vi "Time Shift.vi"(9 "Numeric":i32, 11 "Graph in":cluster{dbl[], dbl[]}) -> (3 "Graph out":cluster{dbl[], dbl[]})   [LabVIEW 2015]
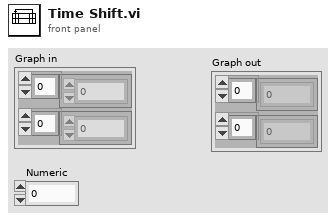
[diagram p1: front panel]
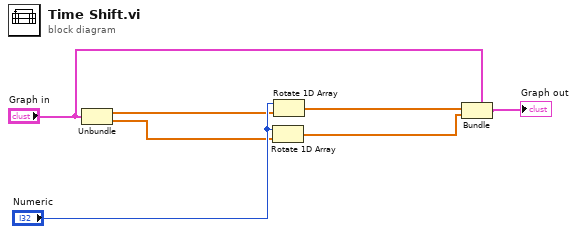
[diagram p0: block diagram]
diagram:
  n1 = Unbundle("Graph in") -> (w6:dbl[], w5:dbl[])
  n2 = Rotate 1D Array(1:w5, 2:"Numeric") -> (0:w2:dbl[])
  n3 = Rotate 1D Array(1:w6, 2:"Numeric") -> (0:w3:dbl[])
  n4 = Bundle(cluster="Graph in", w3, w2) -> (→"Graph out":cluster{dbl[], dbl[]})
